vi "Coord window-Zoom picture map.vi"(11 "Function":enum16{"Zoom in", "Zoom out"}(ring)) -> ()   [LabVIEW 2017]
uses:
  Globals/Coord window-Globals.vi
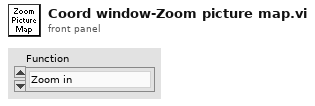
[diagram p1: front panel]
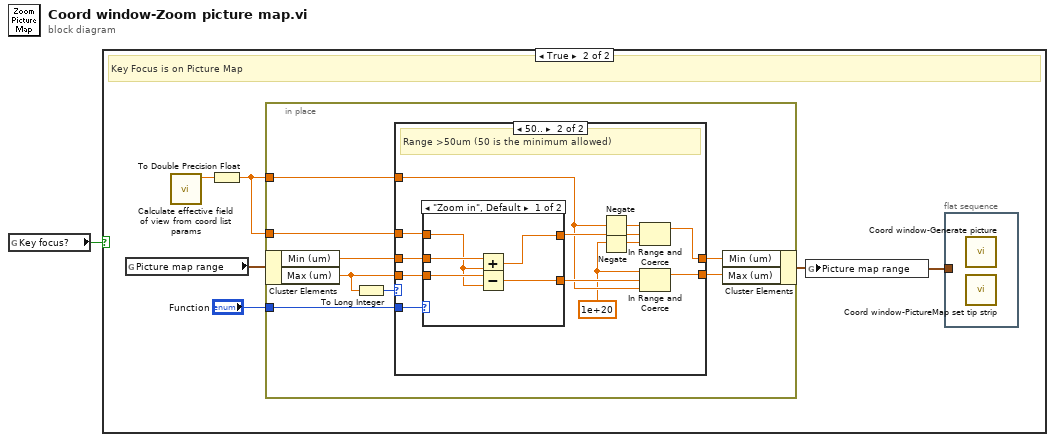
[diagram p0: block diagram]
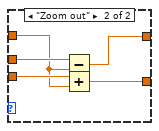
[diagram p4: hidden frame]
diagram:
  n1 = global read "Coord window-Globals.vi" "Key focus?"() -> (w1:bool)
  n2 = case shown="True" w1 {
    frame False {
    }
    frame True {
      # "Key Focus is on Picture Map"
      n3 = global read "Coord window-Globals.vi" "Picture map range"() -> (w5:cluster{"Min (um)":dbl, "Max (um)":dbl})
      n4 = call "Calculate effective field of view from coord list params.vi"() -> ("Effective FOV (um)"=w2:sgl)  [unwired: 11 in]
      n5 = To Double Precision Float(number=w2) -> (double precision float=w4:dbl)
      n6 = in-place {
        in-place-border: "Function" -> [w14]
        in-place-border: w4 -> [w13]
        in-place-border: w4 -> [w9]
        n7 = in-place-cluster #1(w5) -> ("Min (um)"=w10:dbl, "Max (um)"=w8:dbl)
        n8 = To Long Integer(number=w8) -> (32bit integer=w7:i32)
        n9 = case shown="50.." w7 {
          tunnel: w14 -> [_ w28]
          tunnel: w10 -> [w16 w27]
          tunnel: w8 -> [w15 w26]
          tunnel: w13 -> [_ w25]
          tunnel: [w16 w23] -> w12
          tunnel: [w15 w17] -> w11
          tunnel: w9 -> [_ w21]
          frame Default {
            # "Range <50um (50 is the minimum allowed)"
          }
          frame 50.. {
            w18 = 1e+20 ("lower limit")
            # "Range >50um (50 is the minimum allowed)"
            n10 = case shown="\"Zoom in\", Default" w28 {
              tunnel: w27 -> [w33 w38]
              tunnel: w26 -> [w32 w37]
              tunnel: w25 -> [w31 w36]
              tunnel: [w30 w35] -> w24
              tunnel: [w29 w34] -> w22
              frame "Zoom in", Default {
                n11 = Add(x=w33, y=w31) -> (x+y=w30:dbl)
                n12 = Subtract(x=w32, y=w31) -> (x-y=w29:dbl)
              }
              frame "Zoom out" {
                n13 = Subtract(x=w38, y=w36) -> (x-y=w35:dbl)
                n14 = Add(x=w37, y=w36) -> (x+y=w34:dbl)
              }
            }
            n15 = Negate(x=w21) -> (-x=w20:dbl)
            n16 = Negate(x=w18) -> (-x=w19:dbl)
            n17 = In Range and Coerce(upper limit=w20, x=w24, lower limit=w19) -> (coerced(x)=w23:dbl)  [unwired: 1 out]
            n18 = In Range and Coerce(upper limit=w18, x=w22, lower limit=w21) -> (coerced(x)=w17:dbl)  [unwired: 1 out]
          }
        }
        n19 = in-place-cluster #1("Min (um)"=w12, "Max (um)"=w11) -> (w3:cluster{"Min (um)":dbl, "Max (um)":dbl})
      }
      n20 = global write "Coord window-Globals.vi" "Picture map range"(w3) -> ()
      n21 = flat-sequence {
        tunnel: w3 -> [_]
        frame #0 {
          n22 = call "Coord window-Generate picture.vi"() -> ()  [unwired: 11 in, 1 out]
          n23 = call "Coord window-PictureMap set tip strip.vi"() -> ()  [unwired: 12 in]
        }
      }
    }
  }
